vi "BotSpeak_PWM.vi"(0 "Strength (100)":sgl=100.0, 2 "Bot Settings":T1, 3 "PWM Line":u8=3) -> (1 "response":string="Error", 4 "Bot Settings out":T1)   [LabVIEW 2012]
doc: "Uses pulse width modulation to vary the voltage sent out the specified \"DIO Line\". \"Strength\" ranges from 0 to 100, and is a precentage of the max voltage that can be sent through the specified line."
uses:
  <userlib>/BotSpeak/VIs/Direct/BotSpeak_Control.ctl
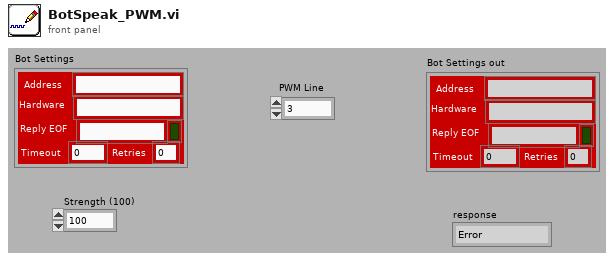
[diagram p1: front panel]
types:
  T1 = typedef "BotSpeak_Control.ctl" = cluster{"Address":string, "Reply EOF":string, "Hardware":string, "Retries":i8, "Timeout":i32, "Open?":bool}
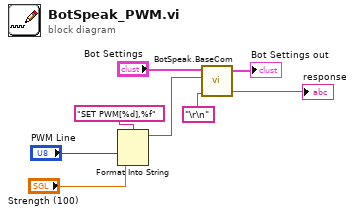
[diagram p0: block diagram]
diagram:
  n1 = Format Into String(format string="SET PWM[%d],%f" ("command"), "PWM Line", "Strength (100)") -> (resulting string=w8:string)  [unwired: 2 in, 1 out]
  n2 = call <userlib>:"BotSpeak.BaseCom.vi"("Termination"="\r\n", "command"=w8, "Bot Settings in"="Bot Settings") -> ("response"=→"response":string, "Bot Settings out"=→"Bot Settings out":T1)  [unwired: 2 in]
